vi "Read NumBytes.vi"(8 "error in (no error)":errorcluster, 11 "Serial Message in":refnum<class "Serial Message.lvclass">) -> (0 "error out":errorcluster, 2 "NumBytes":u8, 3 "Serial Message out":refnum<class "Serial Message.lvclass">)   [LabVIEW 2013, in "Serial Message.lvclass"]
uses:
  Serial Message.lvclass
  Serial Message.lvclass/Serial Message.ctl
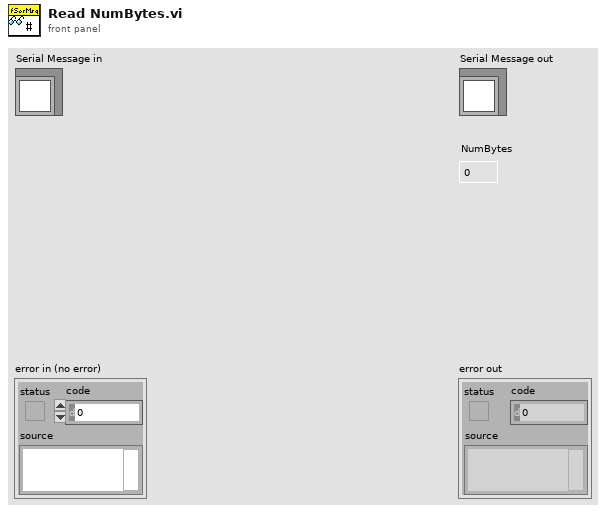
[diagram p1: front panel]
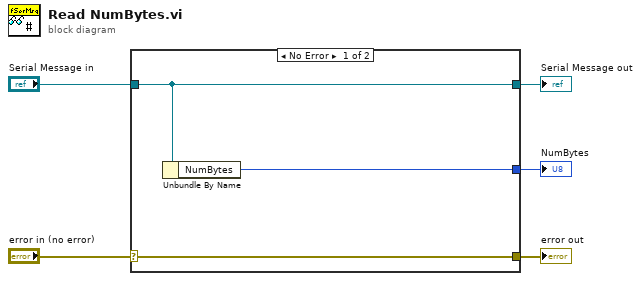
[diagram p0: block diagram]
diagram:
  n1 = case shown="No Error" "error in (no error)" {
    selector: "error in (no error)" -> [w8 w9]
    tunnel: [w8 w9] -> w4
    tunnel: [w7 w10] -> w2
    tunnel: "Serial Message in" -> [w7 w10]
    tunnel: [w6 _] -> w1
    frame No Error {
      n2 = Unbundle By Name(w7) -> ("NumBytes"=w6:u8)
    }
    frame Error {
    }
  }
  "error out" <- w4
  "Serial Message out" <- w2
  "NumBytes" <- w1
